vi "Get Parent.vi"(8 "error in (no error)":errorcluster, 10 "tag":string, 11 "TreeControl in":refnum<vi>) -> (0 "error out":errorcluster, 1 "parent name":string, 2 "parent tag":string, 3 "TreeControl out":refnum<vi>)   [LabVIEW 2017, in "DSF Mini Explorer.lvlib"]
uses:
  DSF Mini Explorer.lvlib
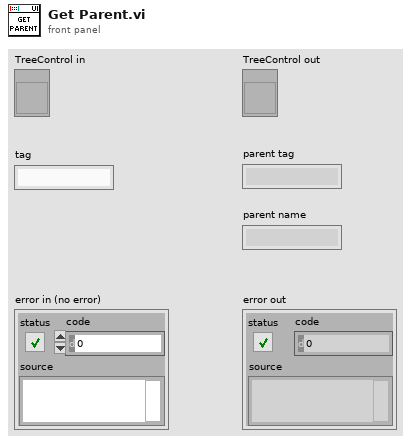
[diagram p1: front panel]
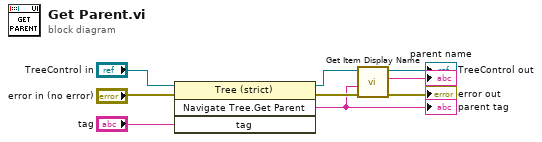
[diagram p0: block diagram]
diagram:
  n1 = invoke class="Tree (strict)" method="Navigate Tree.Get Parent"(reference="TreeControl in", error in="error in (no error)", "tag"="tag") -> (reference out=w8:refnum<vi>, error out=w5:errorcluster, "Navigate Tree:Get Parent"=w4:string)  [unwired: 1 in, 1 out]
  "parent tag" <- w4
  n2 = call "Get Item Display Name.vi"("error in (no error)"=w5, "Tag"=w4, "TreeControl in"=w8) -> ("error out"=→"error out":errorcluster, "display name"=→"parent name":string, "TreeControl out"=→"TreeControl out":refnum<vi>)  [unwired: 6 in]
